vi "detektoranzeige.vi"() -> ()   [LabVIEW 2010]
panel:
  in  "Automatische Skalierung":bool
  in  "Detektor-Nummer":enum16{"0", "1"}(ring)=enum."1"
  in  "Y-Achse:Minimum":dbl
  in  "Y-Achse:Maximum":dbl
  in  "Stopp":bool
  out "Signal":cluster{i32[], i32[]}[](graph)
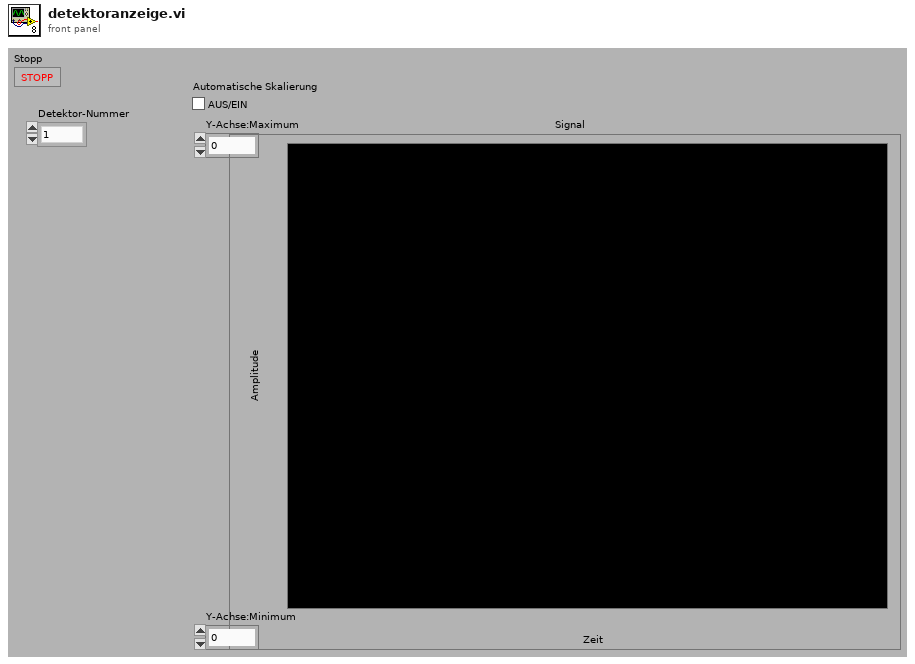
[diagram p1: front panel]
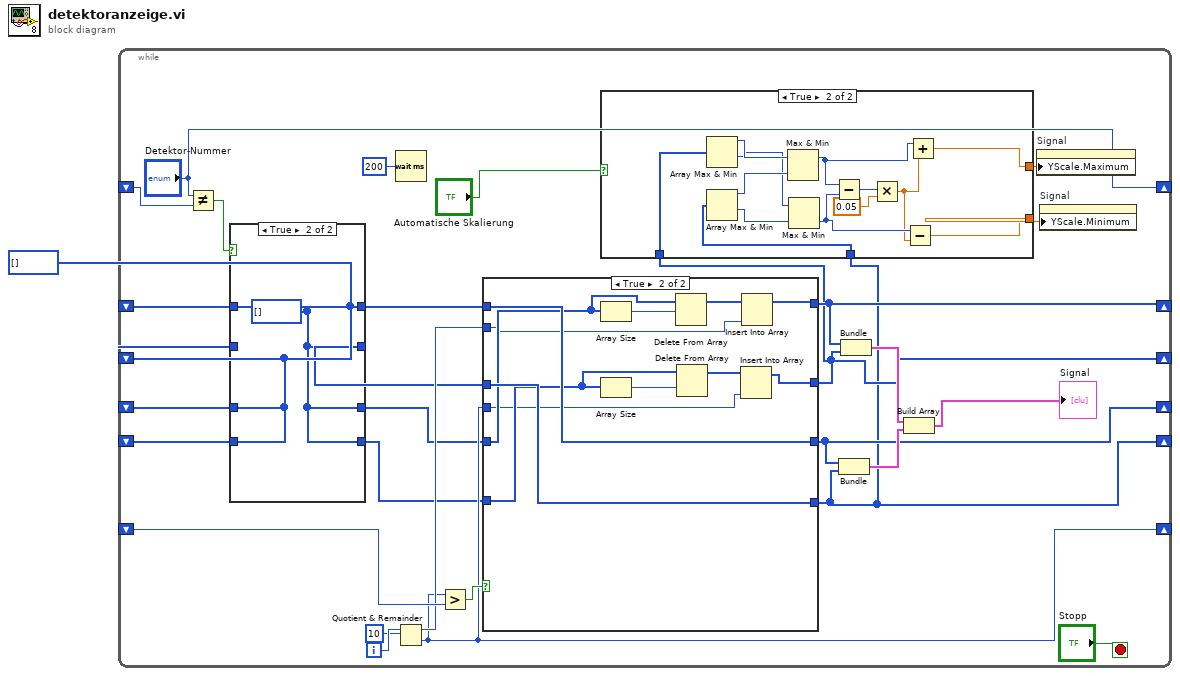
[diagram p0: block diagram]
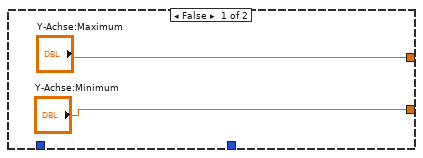
[diagram p2: hidden frame]
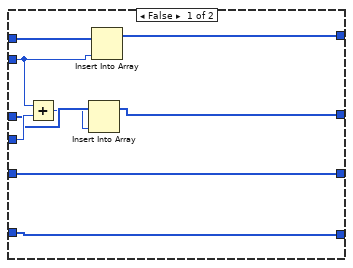
[diagram p4: hidden frame]
diagram:
  w1 = i32[] []
  n1 = while {
    shift-right: [w3] -> _
    shift-left: w1 -> [w15]
    shift-right: [w2] -> _
    shift-left: w1 -> [w11]
    shift-right: [w18] -> _
    shift-left: _ -> [w26]
    shift-right: [w22] -> _
    shift-left: w1 -> [w13]
    shift-right: [w20] -> _
    shift-left: w1 -> [w17]
    shift-right: ["Detektor-Nummer"] -> _
    shift-left: _ -> [w8]
    i -> [w28]
    stop <- "Stopp" stop-if-true
    n2 = Not Equal?(x="Detektor-Nummer", y=w8) -> (x != y?=w7:bool)
    n3 = case shown="True" w7 {
      tunnel: [w49 w50] -> w16
      tunnel: w17 -> [w49 _]
      tunnel: [w48 w50] -> w14
      tunnel: w15 -> [w48 _]
      tunnel: w13 -> [w47 _]
      tunnel: [w47 w50] -> w12
      tunnel: w11 -> [w46 _]
      tunnel: [w46 w50] -> w10
      frame False {
      }
      frame True {
        w50 = i32[] []
      }
    }
    n4 = Wait (ms)(milliseconds to wait=u32 200 ("Zu wartende ms")) -> ()  [unwired: 1 out]
    n5 = Quotient & Remainder(x=w28, y=10) -> (x-y*floor(x/y)=w21:i32, floor(x/y)=w18:i32)
    n6 = Greater?(x=w18, y=w26) -> (0:w25:bool)
    n7 = case shown="True" w25 {
      tunnel: w10 -> [w59 w68]
      tunnel: w14 -> [w53 w71]
      tunnel: [w59 w71] -> w2
      tunnel: w12 -> [w58 w69]
      tunnel: w16 -> [w57 w70]
      tunnel: [w58 w70] -> w22
      tunnel: w21 -> [w55 w64]
      tunnel: [w56 w63] -> w20
      tunnel: w18 -> [w54 w61]
      tunnel: [w51 w60] -> w3
      frame False {
        n8 = Add(x=w55, y=w54) -> (x+y=w52:i32)
        n9 = Insert Into Array(array=w53, new element=w52) -> (w51:i32[])  [unwired: 1 in]
        n10 = Insert Into Array(array=w57, new element=w55) -> (w56:i32[])  [unwired: 1 in]
      }
      frame True {
        n11 = Array Size(array=w69) -> (size(s)=w67:i32)
        n12 = Array Size(array=w68) -> (size(s)=w66:i32)
        n13 = Delete From Array(array=w69, length=w67) -> (array with subset deleted=w65:i32[])  [unwired: 1 in, 1 out]
        n14 = Delete From Array(array=w68, length=w66) -> (array with subset deleted=w62:i32[])  [unwired: 1 in, 1 out]
        n15 = Insert Into Array(array=w62, new element=w61) -> (w60:i32[])  [unwired: 1 in]
        n16 = Insert Into Array(array=w65, new element=w64) -> (w63:i32[])  [unwired: 1 in]
      }
    }
    n17 = case shown="True" "Automatische Skalierung" {
      tunnel: ["Y-Achse:Maximum" w36] -> w5
      tunnel: ["Y-Achse:Minimum" w33] -> w4
      tunnel: w3 -> [_ w45]
      tunnel: w2 -> [_ w44]
      frame False {
      }
      frame True {
        n18 = Array Max & Min(array=w45) -> (max value=w43:i32, min value=w41:i32)  [unwired: 2 out]
        n19 = Array Max & Min(array=w44) -> (max value=w42:i32, min value=w40:i32)  [unwired: 2 out]
        n20 = Max & Min(x=w43, y=w42) -> (max(x,y)=w37:i32)  [unwired: 1 out]
        n21 = Max & Min(x=w41, y=w40) -> (min(x,y)=w35:i32)  [unwired: 1 out]
        n22 = Subtract(x=w37, y=w35) -> (x-y=w39:i32)
        n23 = Multiply(x=w39, y=0.05) -> (x*y=w34:dbl)
        n24 = Subtract(x=w35, y=w34) -> (x-y=w33:dbl)
        n25 = Add(x=w37, y=w34) -> (x+y=w36:dbl)
      }
    }
    n26 = Bundle(w22, w2) -> (w24:cluster{i32[], i32[]})  [unwired: 1 in]
    n27 = Bundle(w20, w3) -> (w19:cluster{i32[], i32[]})  [unwired: 1 in]
    n28 = Build Array(w19, w24) -> (→"Signal":cluster{i32[], i32[]}[])
    n29 = property on="Signal" class="XYGraph (strikt)"("YScale.Maximum"=w5) -> ()  [unwired: 2 in, 2 out]
    n30 = property on="Signal" class="XYGraph (strikt)"("YScale.Minimum"=w4) -> ()  [unwired: 2 in, 2 out]
  }
